vi "Get Control Ref By Class Name.vi"(8 "error in (no error)":errorcluster, 10 "Control Class":string(combo), 11 "[V] Main UI in":refnum<class "[V] Main UI.lvclass">) -> (0 "error out":errorcluster, 2 "refs":refnum<vi>[](array[refnum]), 3 "[V] Main UI out":refnum<class "[V] Main UI.lvclass">)   [LabVIEW 2020, in "[V] Main UI.lvlib" / "[V] Main UI.lvclass"]
uses:
  [V] Main UI.lvclass
  Depden On/Abstruct View/Abstruct View/Abstruct View.lvclass/Abstruct View.ctl
  Depden On/Abstruct View/Abstruct View/Data Accessors/Read Core VI.vi
panel:
  out "Array":string[](array[string])
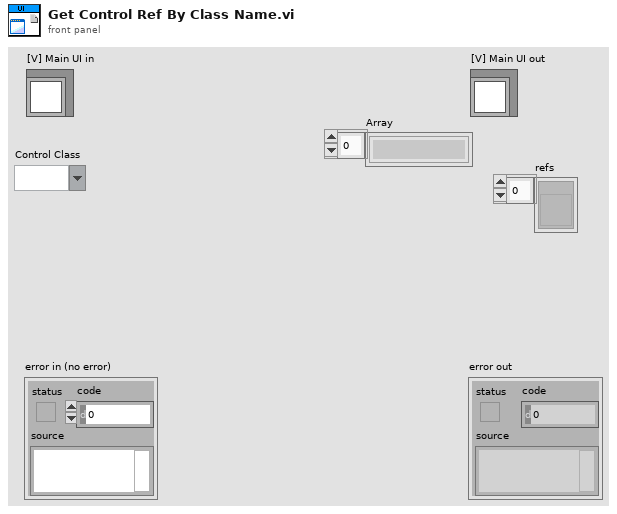
[diagram p1: front panel]
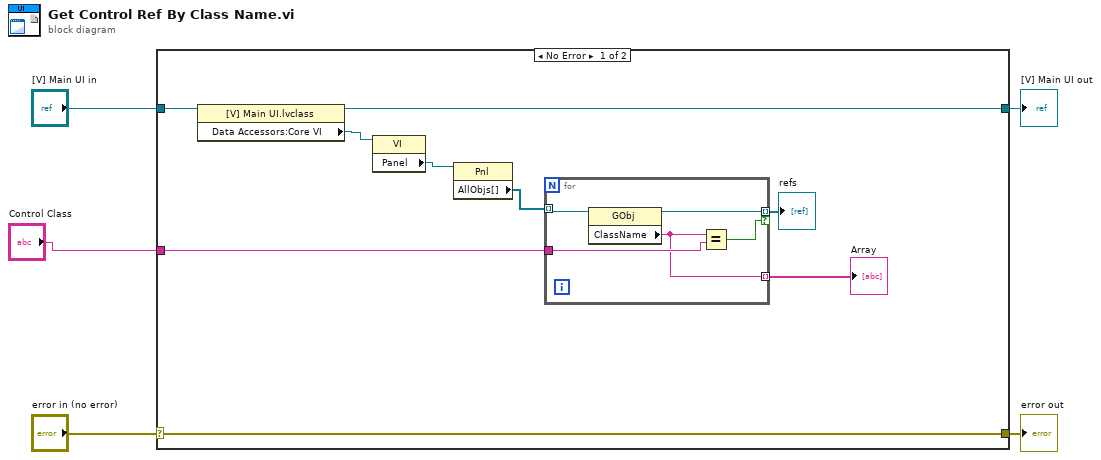
[diagram p0: block diagram]
diagram:
  n1 = case shown="No Error" "error in (no error)" {
    selector: "error in (no error)" -> [w14 w21]
    tunnel: [w14 w21] -> w4
    tunnel: [w12 w20] -> w2
    tunnel: "[V] Main UI in" -> [w13 w20]
    tunnel: "Control Class" -> [w7 _]
    frame No Error {
      n2 = property class="[V] Main UI.lvclass"(reference=w13) -> (reference out=w12:refnum<class "[V] Main UI.lvclass">, "Data Accessors:Core VI"=w9:refnum<vi>)  [unwired: 1 in, 1 out]
      n3 = property class="VI"(reference=w9) -> ("Panel"=w11:refnum<vi>)  [unwired: 1 in, 2 out]
      n4 = property class="Pnl"(reference=w11) -> ("AllObjs[]"=w10:refnum<vi>[])  [unwired: 1 in, 2 out]
      n5 = for {
        tunnel: w10 -> [w19] mode=indexing
        tunnel: [w18] -> w8 mode=indexing if=w17
        tunnel: w7 -> [w16]
        tunnel: [w15] -> w6 mode=indexing
        n6 = property class="GObj"(reference=w19) -> (reference out=w18:refnum<vi>, "ClassName"=w15:string)  [unwired: 1 in, 1 out]
        n7 = Equal?(x=w15, y=w16) -> (x = y?=w17:bool)
      }
      "refs" <- w8
      "Array" <- w6
    }
    frame Error {
    }
  }
  "error out" <- w4
  "[V] Main UI out" <- w2
